vi "ZufälligeTemperatur.vi"   [LabVIEW 2018]
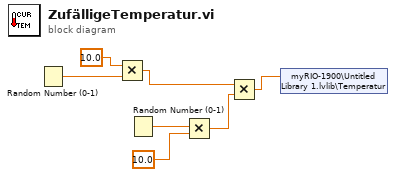
[diagram p0: block diagram]
diagram:
  n1 = Random Number (0-1)() -> (number: 0 to 1=w7:dbl)
  n2 = Multiply(x=10.0, y=w7) -> (x*y=w5:dbl)
  n3 = Random Number (0-1)() -> (number: 0 to 1=w4:dbl)
  n4 = Multiply(x=w4, y=10.0) -> (x*y=w3:dbl)
  n5 = Multiply(x=w5, y=w3) -> (x*y=w2:dbl)
  n6 = shared-variable "myRIO-1900\\Untitled Library 1.lvlib\\Temperatur"(w2) -> ()  [unwired: 1 in, 1 out]
